vi "Grid Settle Timer.vi"(8 "error in (no error)":errorcluster, 11 "IED in":refnum<class "IED.lvclass">) -> (0 "error out":errorcluster, 3 "IED out":refnum<class "IED.lvclass">)   [LabVIEW 2015, in "IED Actor.lvlib" / "IED.lvclass"]
uses:
  IED.lvclass
panel:
  out "Progress":i32(slide) scale=0.0..100.0
  # "Waiting for Grid Settling"
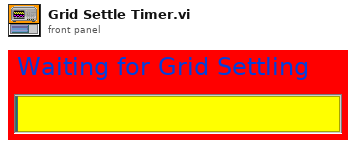
[diagram p1: front panel]
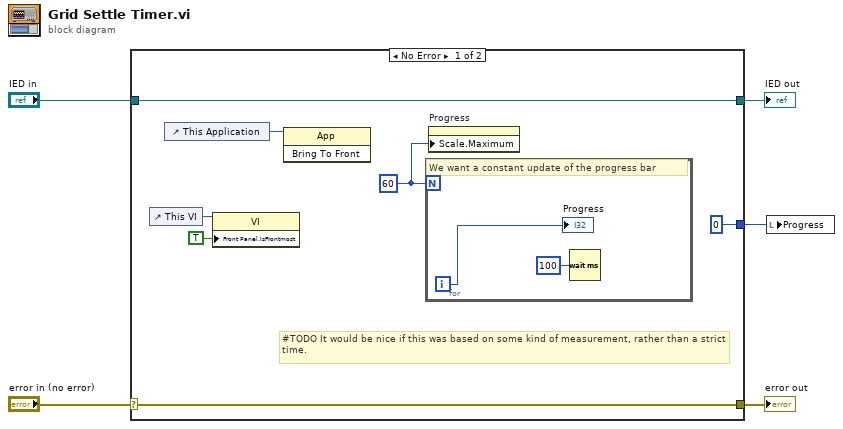
[diagram p0: block diagram]
diagram:
  n1 = case shown="No Error" "error in (no error)" {
    selector: "error in (no error)" -> [w11 w16]
    tunnel: [w11 w16] -> w4
    tunnel: [w12 w15] -> w2
    tunnel: "IED in" -> [w12 w15]
    tunnel: [0 ("Progress") _] -> w1
    frame No Error {
      w10 = 60
      # "#TODO It would be nice if this was based on some kind of measurement, rather than a strict time."
      n2 = control-ref of="This VI"() -> (w6:refnum<vi>)
      n3 = control-ref of="This Application"() -> (w8:refnum<vi>)
      n4 = property class="VI"(reference=w6, "Front Panel.IsFrontmost"=TRUE ("Front Panel Window:Is Frontmost")) -> ()  [unwired: 1 in, 2 out]
      n5 = invoke class="App" method="Bring To Front"(reference=w8) -> ()  [unwired: 2 in, 3 out]
      n6 = for {
        N: w10 -> [_]
        i -> [w14]
        # "We want a constant update of the progress bar"
        n7 = Wait (ms)(milliseconds to wait=u32 100) -> ()  [unwired: 1 out]
        "Progress" <- w14
      }
      n8 = property on="Progress" class="Slide (strict)"("Scale.Maximum"=w10) -> ()  [unwired: 2 in, 2 out]
    }
    frame Error {
    }
  }
  "error out" <- w4
  "IED out" <- w2
  n9 = local write "Progress"(w1) -> ()
